vi "Untitled 2.vi"() -> ()   [LabVIEW 2020]
uses:
  Subsystems/Climber/Climber_Sequences.ctl
panel:
  out "number":i32
  out "confirm step advance 2":bool
  out "reset current sequence 2":bool
  out "Reset_to_first":bool
  out "confirm sequence advance 2":bool
  in  "finished":bool
  in  "Enum":T1
  in  "reset current sequence":bool
  in  "confirm step advance":bool
  in  "move step back":bool
  in  "confirm sequence advance":bool
  in  "reset to first sequence":bool
  in  "Controller_Advance_Step":bool
  in  "Reset_Entire_Sequence":bool
  in  "Enable Front Panel Control":bool
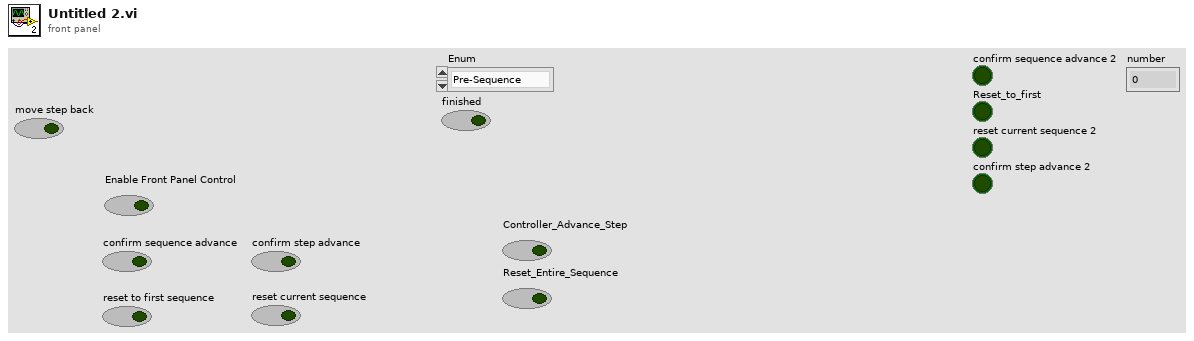
[diagram p1: front panel]
types:
  T1 = typedef "Climber_Sequences.ctl" = enum16{"Pre-Sequence", "Main Sequence"}
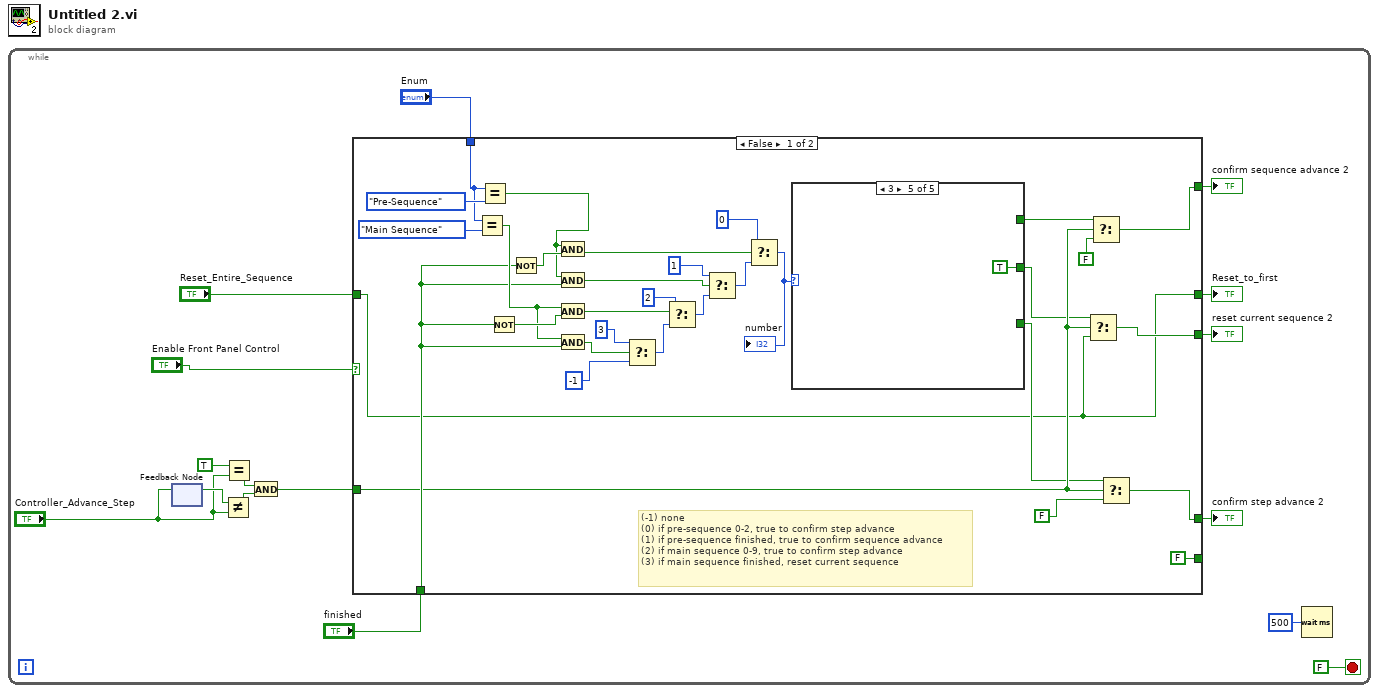
[diagram p0: block diagram]
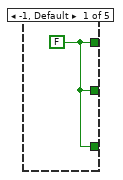
[diagram p2: hidden frame]
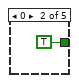
[diagram p3: hidden frame]
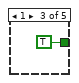
[diagram p4: hidden frame]
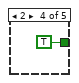
[diagram p5: hidden frame]
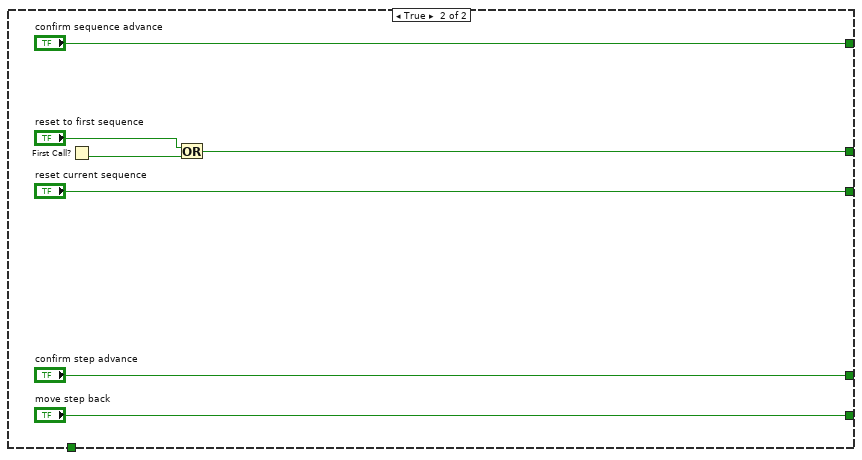
[diagram p6: hidden frame]
diagram:
  n1 = while {
    stop <- FALSE stop-if-true
    n2 = feedback #1() -> (w14:bool)  [unwired: 1 in]
    n3 = feedback-in #1("Controller_Advance_Step") -> ()
    n4 = Not Equal?(x=w14, y="Controller_Advance_Step") -> (x != y?=w10:bool)
    n5 = Equal?(x=TRUE, y="Controller_Advance_Step") -> (x = y?=w11:bool)
    n6 = And(x=w11, y=w10) -> (x .and. y?=w9:bool)
    n7 = case shown="False" "Enable Front Panel Control" {
      tunnel: [w26 "reset current sequence"] -> w4
      tunnel: [w22 "confirm step advance"] -> w3
      tunnel: [FALSE ("move step back") "move step back"] -> _
      tunnel: [w19 "confirm sequence advance"] -> w6
      tunnel: [w17 w54] -> w5
      tunnel: "Reset_Entire_Sequence" -> [w17 _]
      tunnel: w9 -> [w27 _]
      tunnel: "Enum" -> [w45 _]
      tunnel: "finished" -> [w41 _]
      frame False {
        # "(-1) none\n(0) if pre-sequence 0-2, true to confirm step advance\n(1) if pre-sequence finished, true to confirm sequence advance\n(2) if main sequence 0-9, true to confirm step advance\n(3) if main sequence finished, reset current sequence"
        n8 = Equal?(x=w45, y=Climber_Sequences."Main Sequence") -> (x = y?=w42:bool)
        n9 = Equal?(x=w45, y=Climber_Sequences."Pre-Sequence") -> (x = y?=w46:bool)
        n10 = Not(x=w41) -> (.not. x?=w43:bool)
        n11 = Not(x=w41) -> (.not. x?=w47:bool)
        n12 = And(x=w46, y=w47) -> (x .and. y?=w30:bool)
        n13 = And(x=w46, y=w41) -> (x .and. y?=w33:bool)
        n14 = And(x=w42, y=w43) -> (x .and. y?=w36:bool)
        n15 = And(x=w42, y=w41) -> (x .and. y?=w38:bool)
        n16 = Select(t=3, s=w38, f=-1) -> (s? t:f=w37:i32)
        n17 = Select(t=2, s=w36, f=w37) -> (s? t:f=w34:i32)
        n18 = Select(t=1, s=w33, f=w34) -> (s? t:f=w31:i32)
        n19 = Select(t=0, s=w30, f=w31) -> (s? t:f=w28:i32)
        "number" <- w28
        n20 = case shown="3" w28 {
          tunnel: [w49 _ TRUE _ _] -> w20
          tunnel: [w49 _ _ _ TRUE] -> w21
          tunnel: [w49 TRUE _ TRUE _] -> w23
          frame -1, Default {
            w49 = FALSE
          }
          frame 0 {
          }
          frame 1 {
          }
          frame 2 {
          }
          frame 3 {
          }
        }
        n21 = Select(t=w21, s=w27, f=w17) -> (s? t:f=w26:bool)
        n22 = Select(t=w20, s=w27, f=FALSE) -> (s? t:f=w19:bool)
        n23 = Select(t=w23, s=w27, f=FALSE) -> (s? t:f=w22:bool)
      }
      frame True {
        n24 = First Call?() -> (First Call?: T/F=w55:bool)
        n25 = Or(x="reset to first sequence", y=w55) -> (x .or. y?=w54:bool)
      }
    }
    "confirm sequence advance 2" <- w6
    "Reset_to_first" <- w5
    "reset current sequence 2" <- w4
    "confirm step advance 2" <- w3
    n26 = Wait (ms)(milliseconds to wait=u32 500) -> ()  [unwired: 1 out]
  }
